vi "MoveInc.vi"   [LabVIEW 2021]
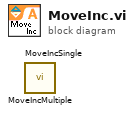
[diagram p0: block diagram]
diagram:
  n1 = call "MoveIncMultiple.vi"() -> ()  [unwired: 10 in, 2 out]
  n2 = call "MoveIncSingle.vi"() -> ()  [unwired: 10 in, 2 out]
